vi "Input Path.vi"() -> (3 "input path":path)   [LabVIEW 2021, in "AOC.lvlib"]
uses:
  AOC.lvlib
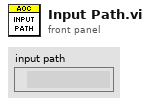
[diagram p1: front panel]
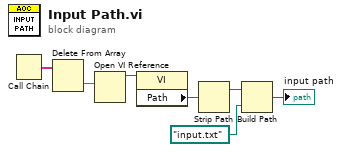
[diagram p0: block diagram]
diagram:
  n1 = Call Chain() -> (call chain=w4:string[])
  n2 = Delete From Array(array=w4) -> (deleted portion=w1:string)  [unwired: 2 in, 1 out]
  n3 = Open VI Reference(vi path=w1) -> (vi reference=w3:refnum<vi>)  [unwired: 5 in, 1 out]
  n4 = property class="VI"(reference=w3) -> ("Path"=w2:path)  [unwired: 1 in, 2 out]
  n5 = Strip Path(path=w2) -> (stripped path=w5:path)  [unwired: 1 out]
  n6 = Build Path(base path=w5, name or relative path=path "input.txt") -> (appended path=→"input path":path)
